vi "Command (read & write) - AC.vi"(7 "timeout ms (100)":i32=100, 8 "error in (no error)":errorcluster, 9 "Acceleration":dbl=-9999.0, 10 "IP":string, 11 "connection ID in":refnum<k16>) -> (0 "error out":errorcluster, 2 "Acceleration":dbl, 3 "connection ID out":refnum<k16>)   [LabVIEW 2016, in "SMD-7615.lvlib" / "eSCL.lvlib"]
doc: "AC - Acceleration Rate\nSets or requests the acceleration rate used in point-to-point move commands in rev/sec/sec."
uses:
  eSCL.lvlib
  DBL Command and Param.ctl
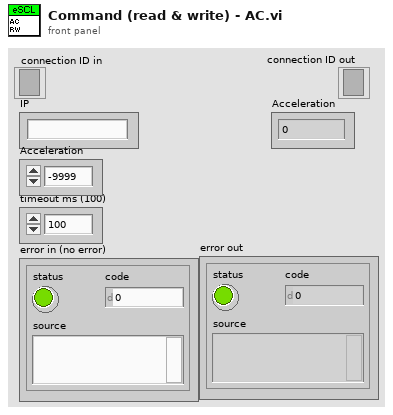
[diagram p1: front panel]
types:
  T1 = typedef "SMD-7615.lvlib/eSCL.lvlib/DBL Command and Param.ctl" = cluster{"Command":string, "DBL Parameler":dbl, "DBL Parameler Default":dbl, "DBL Parameler Coerece Upper":dbl, "DBL Parameler Coerece Lower":dbl}
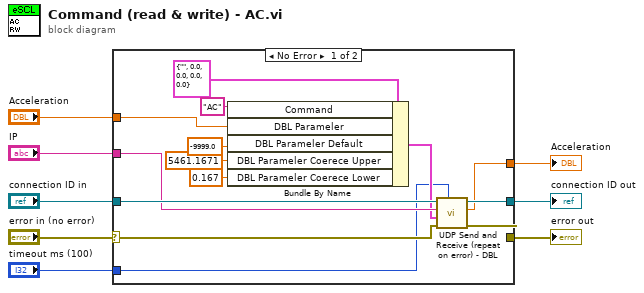
[diagram p0: block diagram]
diagram:
  n1 = case shown="No Error" "error in (no error)" {
    selector: "error in (no error)" -> [w13 w23]
    tunnel: "connection ID in" -> [w16 w24]
    tunnel: [w11 w24] -> w6
    tunnel: [w10 w23] -> w5
    tunnel: "IP" -> [w15 _]
    tunnel: "timeout ms (100)" -> [w12 _]
    tunnel: [w9 _] -> w2
    tunnel: "Acceleration" -> [w17 _]
    frame No Error {
      n2 = Bundle By Name(cluster=T1 {"Command"="", "DBL Parameler"=0.0, "DBL Parameler Default"=0.0, "DBL Parameler Coerece Upper"=0.0, "DBL Parameler Coerece Lower"=0.0} ("DBL Command & Param"), "Command"="AC", "DBL Parameler"=w17, "DBL Parameler Default"=-9999.0, "DBL Parameler Coerece Upper"=5461.1671, "DBL Parameler Coerece Lower"=0.167) -> (w14:T1)
      n3 = call "UDP Send and Receive (repeat on error) - DBL.vi"("timeout ms (100)"=w12, "error in (no error)"=w13, "DBL Command & Param"=w14, "IP"=w15, "connection ID in"=w16) -> ("error out"=w10:errorcluster, "DBL Param out"=w9:dbl, "connection ID out"=w11:refnum<k16>)  [unwired: 4 in]
    }
    frame Error {
    }
  }
  "connection ID out" <- w6
  "error out" <- w5
  "Acceleration" <- w2
